vi "Memory.Pointer.Byte Order.vi"(8 "error in (no error)":errorcluster) -> (0 "error out":errorcluster, 2 "Host byte order":T1, 3 "LabVIEW byte order":T1)   [LabVIEW 2016, in "Memory Manager.lvlib" / "Memory.Pointer.lvclass"]
uses:
  Memory.Pointer.lvclass
  Typedefs/Memory.Pointer.Byte Order.ctl
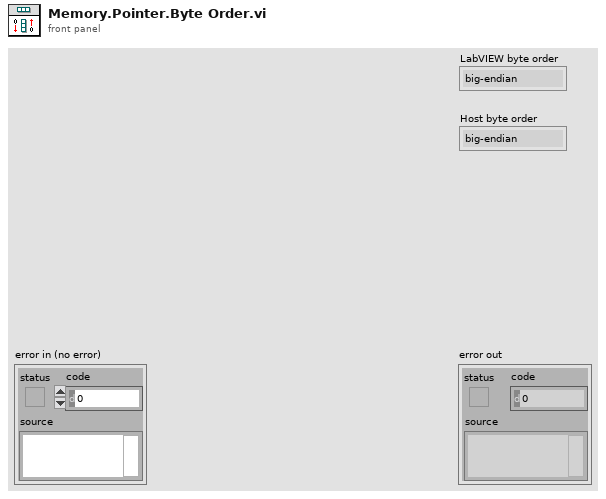
[diagram p1: front panel]
types:
  T1 = typedef "Memory Manager.lvlib/Memory.Pointer.lvclass/Memory.Pointer.Byte Order.ctl" = enum8{"big-endian", "little-endian"}
  T2 = enum16{"big-endian, network order", "native, host order", "little-endian"}
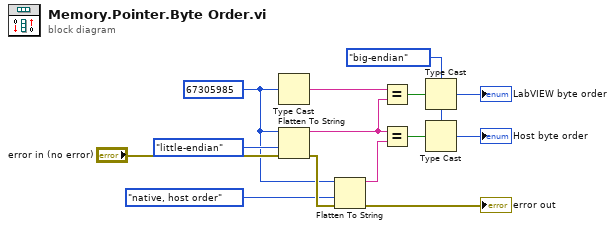
[diagram p0: block diagram]
diagram:
  w4 = Memory.Pointer.Byte_Order."big-endian" ("byte order")
  w7 = u32 67305985
  n1 = Type Cast(x=w7) -> (*(type *) &x=w10:string)  [unwired: 1 in]
  n2 = Flatten To String(anything=w7, byte order (0:big-endian, network order)=T2."little-endian", error in (no error)="error in (no error)") -> (data string=w9:string, error out=w14:errorcluster)  [unwired: 1 in, 1 out]
  n3 = Flatten To String(anything=w7, byte order (0:big-endian, network order)=T2."native, host order", error in (no error)=w14) -> (data string=w8:string, error out=→"error out":errorcluster)  [unwired: 1 in, 1 out]
  n4 = Equal?(x=w10, y=w9) -> (x = y?=w5:bool)
  n5 = Equal?(x=w9, y=w8) -> (x = y?=w6:bool)
  n6 = Type Cast(type=w4, x=w5) -> (*(type *) &x=→"LabVIEW byte order":T1)
  n7 = Type Cast(type=w4, x=w6) -> (*(type *) &x=→"Host byte order":T1)
